vi "Write 2-Tier rank.vi"(10 "2-Tier rank":u8, 11 "ProjectItem in":refnum<class "ProjectItem.lvclass">) -> (3 "ProjectItem out":refnum<class "ProjectItem.lvclass">)   [LabVIEW 2019, in "SolutionBuilder.lvlib" / "ProjectItem.lvclass"]
uses:
  ProjectItem.lvclass
  ProjectItem.lvclass/ProjectItem.ctl
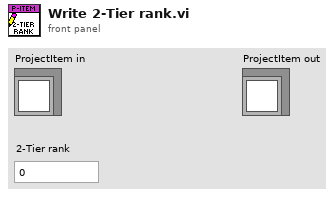
[diagram p1: front panel]
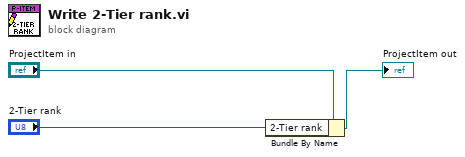
[diagram p0: block diagram]
diagram:
  n1 = Bundle By Name(cluster="ProjectItem in", "2-Tier rank"="2-Tier rank") -> (→"ProjectItem out":refnum<class "ProjectItem.lvclass">)
